vi "Actor Core.vi"(8 "error in":errorcluster, 11 "Manager in":refnum<class "Manager.lvclass">) -> (0 "error out":errorcluster, 3 "Actor out":refnum<class "Actor.lvclass">)   [LabVIEW 2016, in "Manager.lvlib" / "Manager.lvclass"]
doc: "(<B>Filename</B>: Actor Framework.lvlib:Actor.lvclass:Actor Core.vi)\n\nReceives messages to the actor, reacts to them, and initiates any error handling that may shut the actor down.\n\nDescendant classes may override this VI to append parallel tasks for the actor to complete while it handles messages. Overrides use the Call Parent Method node."
uses:
  Manager.lvclass
  C:/Program Files (x86)/National Instruments/LabVIEW 2016/vi.lib/ActorFramework/Actor/Actor.lvclass
  <vilib>/ActorFramework/Actor/Actor.lvclass
  <vilib>/ActorFramework/Actor/Actor.lvclass/Actor.ctl
  <vilib>/ActorFramework/Message Enqueuer/Message Enqueuer.lvclass/Message Enqueuer.ctl
  Manager.lvclass/Manager.ctl
  Service Types.ctl
  Manager Messages/Launch New Service Msg/Launch New Service Msg.lvclass/Launch New Service Msg.ctl
  <vilib>/NI/STM/UDP/UDP Read Options.ctl
  <vilib>/NI/STM/UDP/Read Meta Data (UDP Ref).vi
  <vilib>/NI/STM/UDP/Get Connection Reference (UDP).vi
  <vilib>/ActorFramework/Message Enqueuer/Init from Existing Queue.vi
  <vilib>/ActorFramework/Message Enqueuer/Enqueue.vi
  Manager Messages/Launch New Service Msg/Launch New Service Msg.lvclass
  C:/Program Files (x86)/National Instruments/LabVIEW 2016/vi.lib/ActorFramework/Message/Message.lvclass
  <vilib>/ActorFramework/Stop Msg/Stop Msg.lvclass
  <vilib>/NI/STM/UDP/Read Meta Data (UDP Clst).vi
  <vilib>/ActorFramework/Message Priority Queue/Priority Enqueue.vi
  <vilib>/NI/STM/UDP/Read Message (UDP).vi
  <vilib>/ActorFramework/Message Enqueuer/Message Enqueuer.lvclass
  <vilib>/NI/STM/NI STM.lvlib
panel:
  out "Connected Clients":string[](array[string]) caption="data string"
  in  "New":bool
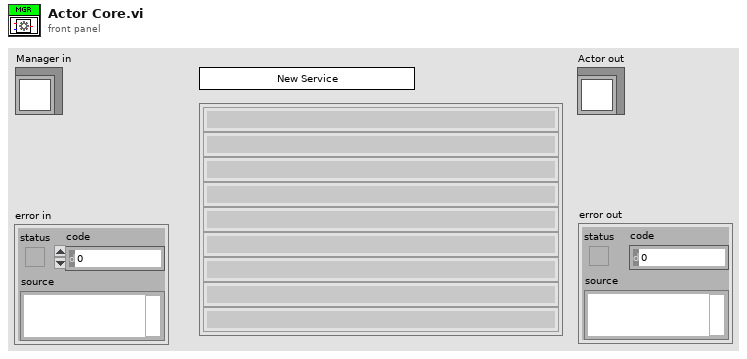
[diagram p1: front panel]
types:
  T1 = typedef "NI STM.lvlib/UDP Connection Info.ctl" = cluster{"connection ID":refnum<k16>, "meta data":T2[]}
  T2 = typedef "NI STM.lvlib/MetaDataElement.ctl" = string
  T3 = typedef "Manager.lvlib/Manager.lvclass/Service Types.ctl" = enum16{"Client", "Server"}
  T4 = typedef "NI STM.lvlib/UDP Read Options.ctl" = cluster{"ignore timeout error":bool, "timeout ms (1000)":i32, "max size (548)":i32}
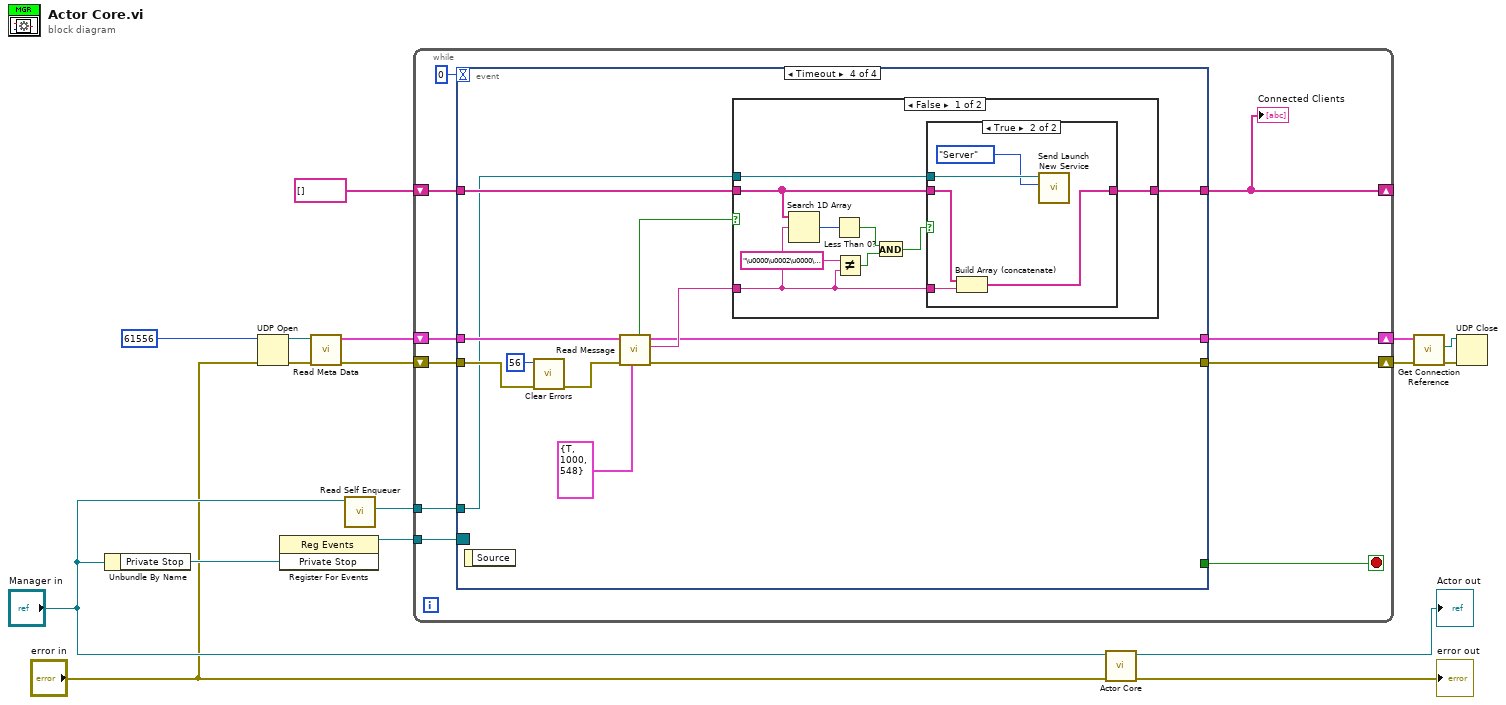
[diagram p0: block diagram]
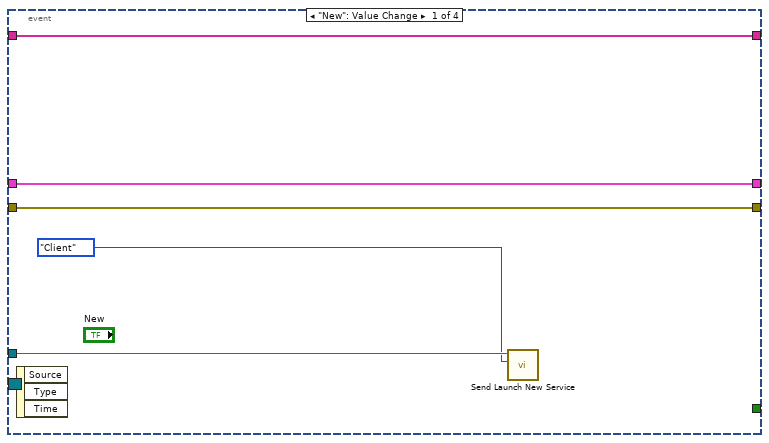
[diagram p2: hidden frame]
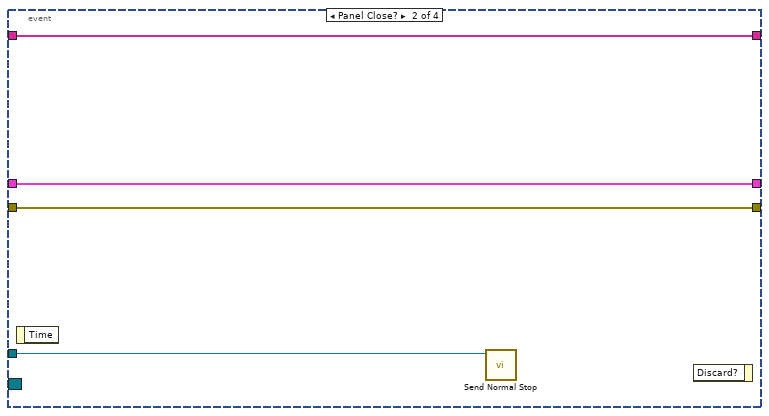
[diagram p3: hidden frame]
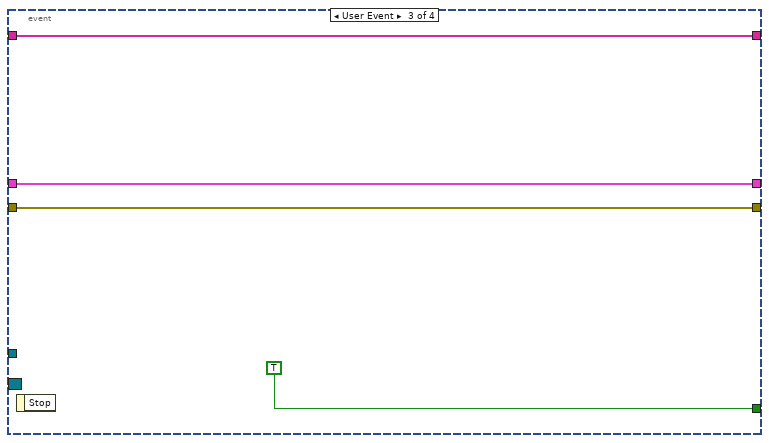
[diagram p4: hidden frame]
diagram:
  n1 = Unbundle By Name("Manager in") -> ("Private Stop"=w13:refnum<user-event>)
  n2 = UDP Open(8:"error in", 11:u16 61556 ("local port")) -> (port=w4:refnum<k16>, 0:w11:errorcluster)  [unwired: 4 out]
  n3 = register-events(w13) -> (reference out=w12:refnum<event-registration>)  [unwired: 2 in, 1 out]
  n4 = call-poly <vilib>:"Read Meta Data.vi"("error in"=w11, "connection ID"=w4) -> ("error out"=w9:errorcluster, "connection info out"=w10:T1)  [unwired: 6 in, 2 out]
  n5 = call <vilib>:"Read Self Enqueuer.vi"("Actor"="Manager in") -> ("Self Enqueuer"=w15:refnum<class "Message Enqueuer.lvclass">)  [unwired: 10 in]
  n6 = while {
    tunnel: w15 -> [w27]
    tunnel: w12 -> [w26]
    shift-right: [w21] -> w6
    shift-left: w10 -> [w23]
    shift-right: [w20] -> w7
    shift-left: w9 -> [w22]
    shift-right: [w18] -> _
    shift-left: string[] [] -> [w19]
    stop <- w25 stop-if-true
    n7 = event shown="[3] Timeout" {
      selector: w26 -> [_ _ _ _]
      dyn-events: _ -> [_ _ _ _]
      timeout: 0 -> [_ _ _ _]
      tunnel: w27 -> [w32 w36 _ w41]
      tunnel: [_ _ TRUE _] -> w25
      tunnel: w23 -> [w30 w35 w39 w52]
      tunnel: w22 -> [w29 w34 w38 w51]
      tunnel: [w30 w35 w39 w49] -> w21
      tunnel: [w29 w34 w38 w48] -> w20
      tunnel: w19 -> [w28 w33 w37 w43]
      tunnel: [w28 w33 w37 w42] -> w18
      event "New": Value Change {
        n8 = event-data() -> ()  [unwired: 1 in, 3 out]
        n9 = call "Send Launch New Service.vi"("Service Type"=Service_Types."Client", "Message Enqueuer"=w32) -> ()  [unwired: 8 in, 2 out]
      }
      event Panel Close? {
        n10 = event-data() -> ()  [unwired: 1 in, 1 out]
        n11 = call <vilib>:"Send Normal Stop.vi"("Message Enqueuer"=w36) -> ()  [unwired: 10 in, 1 out]
        n12 = event-data() -> ()  [unwired: 2 in, 1 out]
      }
      event User Event {
        n13 = event-data() -> ()  [unwired: 1 in, 1 out]
      }
      event Timeout {
        n14 = event-data() -> ()  [unwired: 1 in, 1 out]
        n15 = call <vilib>:"Clear Errors.vi"("error in (no error)"=w51, "specific error code to clear (0: all)"=56) -> ("error out"=w46:errorcluster)  [unwired: 4 in, 1 out]
        n16 = call-poly <vilib>:"Read Message.vi"("options"=T4 {"ignore timeout error"=TRUE, "timeout ms (1000)"=1000, "max size (548)"=548}, "error in"=w46, "connection info in"=w52) -> ("error out"=w48:errorcluster, "data string"=w50:string, "connection info out"=w49:T1, "timed out?"=w47:bool)  [unwired: 1 in, 4 out]
        n17 = case shown="False" w47 {
          tunnel: w50 -> [w57 _]
          tunnel: w43 -> [w60 w68]
          tunnel: [w61 w68] -> w42
          tunnel: w41 -> [w59 _]
          frame False {
            n18 = Search 1D Array(1D array=w60, element=w57) -> (index of element=w58:i32)  [unwired: 1 in]
            n19 = Less Than 0?(x=w58) -> (x < 0?=w55:bool)
            n20 = Not Equal?(x="\u0000\u0002\u0000\u0000\u0000\u0002IP\u0000\u0000\u0000\u0003Ack", y=w57) -> (x != y?=w54:bool)
            n21 = And(x=w55, y=w54) -> (x .and. y?=w53:bool)
            n22 = case shown="True" w53 {
              tunnel: [w62 w67] -> w61
              tunnel: w60 -> [w62 w66]
              tunnel: w57 -> [_ w65]
              tunnel: w59 -> [_ w64]
              frame False {
              }
              frame True {
                n23 = Build Array (concatenate)(w66, w65) -> (w67:string[])
                n24 = call "Send Launch New Service.vi"("Service Type"=Service_Types."Server", "Message Enqueuer"=w64) -> ()  [unwired: 8 in, 2 out]
              }
            }
          }
          frame True {
          }
        }
      }
    }
    "Connected Clients" <- w18
  }
  n25 = call-parent "Actor Core.vi"("error in"="error in", "Actor in"="Manager in") -> ("error out"=→"error out":errorcluster, "Actor out"=→"Actor out":refnum<class "Actor.lvclass">)  [unwired: 8 in]
  n26 = call-poly <vilib>:"Get Connection Reference.vi"("error in"=w7, "connection info in"=w6) -> ("error out"=w8:errorcluster, "connection ID"=w3:refnum<k16>)  [unwired: 8 out]
  n27 = UDP Close(connection ID=w3, 8:w8) -> ()  [unwired: 2 out]
